vi "MainScriptCreateAllIOselectors.vi"   [LabVIEW 2023]
uses:
  <vilib>/numeric/LVNumericRepresentation.ctl
panel:
  # "VI for creating by scripting all the FPGA I/O node selectors,\nbased on case structures wrapping individual Element I/Os"
types:
  T1 = typedef "LVNumericRepresentation.ctl" = enum32{"Extended Precision", "Double Precision", "Single Precision", "Long", "Word", "Byte", "Unsigned Long", "Unsigned Word", "Unsigned Byte", "Complex Extended", "Complex Double", "Complex Single", "Quad", "Unsigned Quad", "Fixed-Point"}
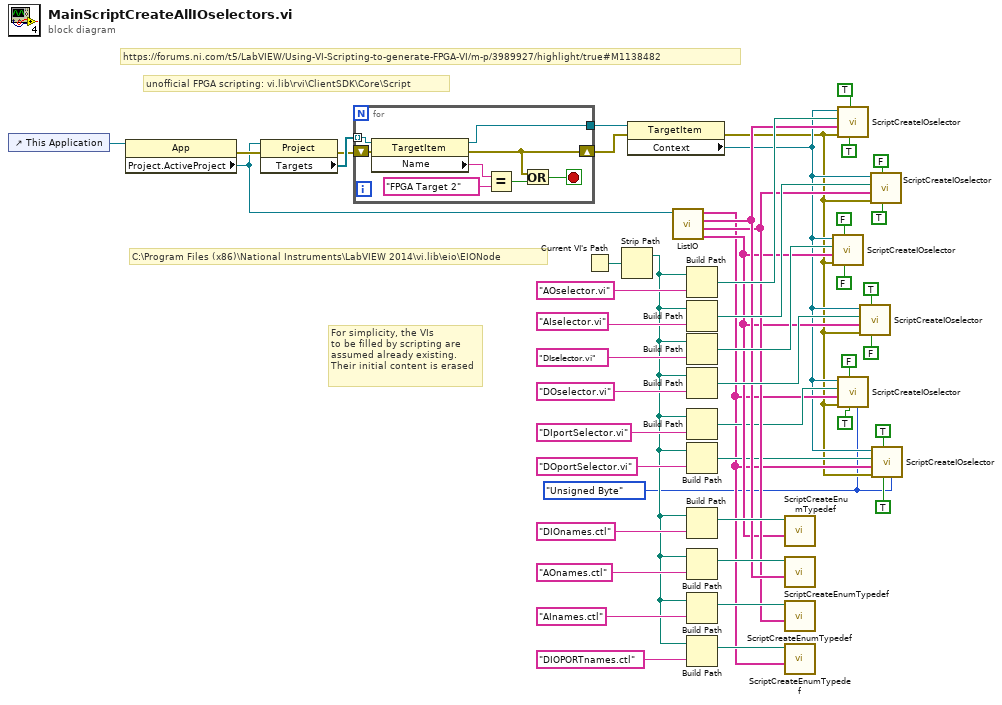
[diagram p0: block diagram]
diagram:
  w1 = LVNumericRepresentation."Unsigned Byte" ("numeric representation")
  # "For simplicity, the VIs\nto be filled by scripting are\nassumed already existing.\nTheir initial content is erased"
  # "C:\\Program Files (x86)\\National Instruments\\LabVIEW 2014\\vi.lib\\eio\\EIONode"
  # "https://forums.ni.com/t5/LabVIEW/Using-VI-Scripting-to-generate-FPGA-VI/m-p/3989927/highlight/true#M1138482"
  # "unofficial FPGA scripting: vi.lib\\rvi\\ClientSDK\\Core\\Script"
  n1 = control-ref of="This Application"() -> (w41:refnum<vi>)
  n2 = property class="App"(reference=w41) -> (error out=w44:errorcluster, "Project.ActiveProject"=w26:refnum<vi>)  [unwired: 1 in, 1 out]
  n3 = property class="Project"(reference=w26, error in=w44) -> (error out=w43:errorcluster, "Targets"=w48:refnum<vi>[])  [unwired: 1 out]
  n4 = for {
    tunnel: w48 -> [w56] mode=indexing
    tunnel: [w53] -> w45
    shift-right: [w49] -> w42
    shift-left: w43 -> [w51]
    stop <- w50 stop-if-true
    n5 = property class="TargetItem"(reference=w56, error in=w51) -> (reference out=w53:refnum<vi>, error out=w49:errorcluster, "Name"=w55:string)
    n6 = Equal?(x=w55, y="FPGA Target 2" ("String")) -> (x = y?=w54:bool)
    n7 = Or(x=w49, y=w54) -> (x .or. y?=w50:bool)
  }
  n8 = Current VI's Path() -> (path=w47:path)
  n9 = Strip Path(path=w47) -> (stripped path=w2:path)  [unwired: 1 out]
  n10 = property class="TargetItem"(reference=w45, error in=w42) -> (error out=w3:errorcluster, "Context"=w4:refnum<vi>)  [unwired: 1 out]
  n11 = call "ListIO.vi"("Project"=w26) -> ("DI/O"=w13:string[], "AI"=w18:string[], "AO"=w19:string[], "DIOPORT"=w5:string[])  [unwired: 7 in]
  n12 = Build Path(base path=w2, name or relative path="AOselector.vi") -> (appended path=w39:path)
  n13 = Build Path(base path=w2, name or relative path="AIselector.vi") -> (appended path=w29:path)
  n14 = Build Path(base path=w2, name or relative path="DIselector.vi") -> (appended path=w32:path)
  n15 = Build Path(base path=w2, name or relative path="DOselector.vi") -> (appended path=w33:path)
  n16 = Build Path(base path=w2, name or relative path="DIportSelector.vi") -> (appended path=w8:path)
  n17 = Build Path(base path=w2, name or relative path="DOportSelector.vi") -> (appended path=w7:path)
  n18 = Build Path(base path=w2, name or relative path="DIOnames.ctl") -> (appended path=w25:path)
  n19 = Build Path(base path=w2, name or relative path="AOnames.ctl") -> (appended path=w22:path)
  n20 = Build Path(base path=w2, name or relative path="AInames.ctl") -> (appended path=w21:path)
  n21 = Build Path(base path=w2, name or relative path="DIOPORTnames.ctl") -> (appended path=w16:path)
  n22 = call "ScriptCreateEnumTypedef.vi"("I/O names"=w13, "Path to Saved File"=w25) -> ()  [unwired: 10 in]
  n23 = call "ScriptCreateEnumTypedef.vi"("I/O names"=w19, "Path to Saved File"=w22) -> ()  [unwired: 10 in]
  n24 = call "ScriptCreateEnumTypedef.vi"("I/O names"=w18, "Path to Saved File"=w21) -> ()  [unwired: 10 in]
  n25 = call "ScriptCreateEnumTypedef.vi"("I/O names"=w5, "Path to Saved File"=w16) -> ()  [unwired: 10 in]
  n26 = call "ScriptCreateIOselector.vi"("digital(F)/numeric(T)"=FALSE, "indicator (F)/control (T)"=FALSE, "error in (no error)"=w3, "IO names"=w13, "VI path"=w32, "Application in"=w4) -> ()  [unwired: 6 in]
  n27 = call "ScriptCreateIOselector.vi"("digital(F)/numeric(T)"=TRUE, "indicator (F)/control (T)"=TRUE, "error in (no error)"=w3, "IO names"=w19, "VI path"=w39, "Application in"=w4) -> ()  [unwired: 6 in]
  n28 = call "ScriptCreateIOselector.vi"("numeric representation"=w1, "digital(F)/numeric(T)"=TRUE, "indicator (F)/control (T)"=FALSE, "error in (no error)"=w3, "IO names"=w5, "VI path"=w8, "Application in"=w4) -> ()  [unwired: 5 in]
  n29 = call "ScriptCreateIOselector.vi"("digital(F)/numeric(T)"=FALSE, "indicator (F)/control (T)"=TRUE, "error in (no error)"=w3, "IO names"=w13, "VI path"=w33, "Application in"=w4) -> ()  [unwired: 6 in]
  n30 = call "ScriptCreateIOselector.vi"("digital(F)/numeric(T)"=TRUE, "indicator (F)/control (T)"=FALSE, "error in (no error)"=w3, "IO names"=w18, "VI path"=w29, "Application in"=w4) -> ()  [unwired: 6 in]
  n31 = call "ScriptCreateIOselector.vi"("numeric representation"=w1, "digital(F)/numeric(T)"=TRUE, "indicator (F)/control (T)"=TRUE, "error in (no error)"=w3, "IO names"=w5, "VI path"=w7, "Application in"=w4) -> ()  [unwired: 5 in]
